vi "실습 9-3 텍스트 파일 읽기.vi"() -> ()   [LabVIEW 2014]
panel:
  out "부분배열":dbl[](array[numeric])
  out "배열":dbl[][](array[numeric])
  out "텍스트":string
  in  "파일 경로(대화 상자 사용)":path
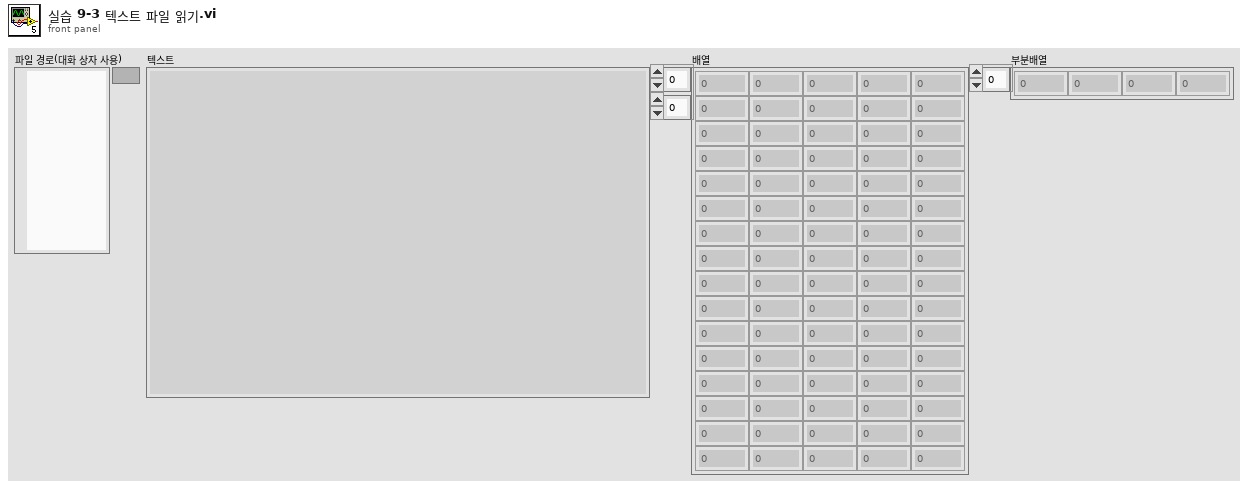
[diagram p1: front panel]
types:
  T1 = enum16{"open", "replace", "create", "open or create", "replace or create", "replace or create with confirmation"}
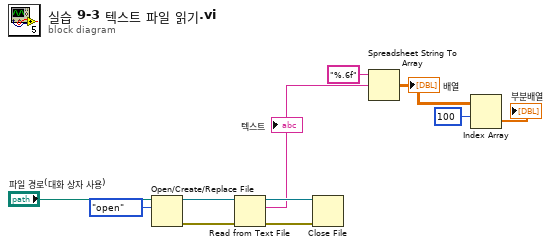
[diagram p0: block diagram]
diagram:
  n1 = Open/Create/Replace File(file path (use dialog)="파일 경로(대화 상자 사용)", operation (0:open)=T1."open" ("동작(0:open)")) -> (refnum out=w11:refnum<file>, error out=w9:errorcluster)  [unwired: 4 in, 1 out]
  n2 = Read from Text File(file (use dialog)=w11, error in=w9) -> (refnum out=w10:refnum<file>, text=w5:string, error out=w8:errorcluster)  [unwired: 2 in, 1 out]
  "텍스트" <- w5
  n3 = Close File(refnum=w10, error in=w8) -> ()  [unwired: 2 out]
  n4 = Spreadsheet String To Array(format string="%.6f" ("포맷 문자열"), spreadsheet string=w5) -> (array=w3:dbl[][])  [unwired: 2 in]
  "배열" <- w3
  n5 = Index Array(array=w3, index (row)=100 ("인덱스 (행)")) -> (element=→"부분배열":dbl[])  [unwired: 1 in]
